vi "Load Setting.vi"(8 "error in (no error)":errorcluster, 11 "Log Config Path":path) -> (0 "error out":errorcluster, 2 "Setting":T1)   [LabVIEW 2020, in "Logging.lvlib"]
uses:
  Logging.lvlib
  Define/Log Setting.ctl
  Define/Logger Setting.ctl
  Define/Log Option.ctl
  Define/Log Level.ctl
  <vilib>/Utility/xml.llb/Read From XML File(string).vi
  Logger Mananger/Logger Mananger.lvclass
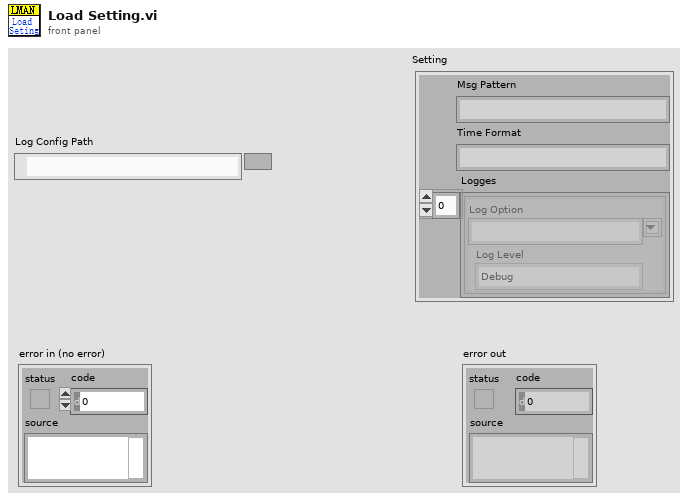
[diagram p1: front panel]
types:
  T1 = typedef "Logging.lvlib/Log Setting.ctl" = cluster{"Msg Pattern":string, "Time Format":string, "Logges":T2[]}
  T2 = typedef "Logging.lvlib/Logger Setting.ctl" = cluster{"Log Option":T3, "Log Level":T4}
  T3 = typedef "Logging.lvlib/Log Option.ctl" = string
  T4 = typedef "Logging.lvlib/Log Level.ctl" = enum16{"Debug", "Info", "Warn", "Error"}
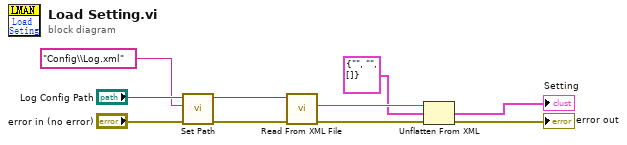
[diagram p0: block diagram]
diagram:
  n1 = call "Set Path.vi"("error in (no error)"="error in (no error)", "Defualt(Sys Relative)"="Config\\Log.xml", "Custom Path"="Log Config Path") -> ("error out"=w2:errorcluster, "Path"=w4:path)  [unwired: 7 in]
  n2 = call-poly <vilib>:"Read From XML File.vi"("error in (no error)"=w2, "XML File Path"=w4) -> ("error out"=w8:errorcluster, "XML Elements"=w10:string)  [unwired: 7 in, 1 out]
  n3 = Unflatten From XML(xml string=w10, type=T1 {"Msg Pattern"="", "Time Format"="", "Logges"=[]} ("Setting"), error in (no error)=w8) -> (value=→"Setting":T1, error out=→"error out":errorcluster)
